vi "LoadFunction.vi"(8 "No Error":errorcluster, 10 "Name":string, 11 "Handle [SDL_SharedObject *]":i64 format="%.0x") -> (0 "Error Out":errorcluster, 3 "Function Pointer":i64 format="%.0x")   [LabVIEW 2024, in "SDL3.lvlib" / "LoadSO.lvlib"]
doc: "<B>Summary</B>\nLook up the address of the named function in a shared object.\n\n<B>Remarks</B>\nThis function pointer is no longer valid after calling <B>SDL_UnloadObject()</B>.\n\nThis function can only look up C function names. Other languages may have name mangling and intrinsic language support that varies from compiler to compiler.\n\nMake sure you declare your function pointers with the same calling convention as the actual library function. Your code will crash mysteriously if you do not do this.\n\nIf the requested function doesn't exist, NULL is returned."
uses:
  LoadSO/LoadSO.lvlib
  Error/Error.lvlib
  Lib/SDL3-32.dll
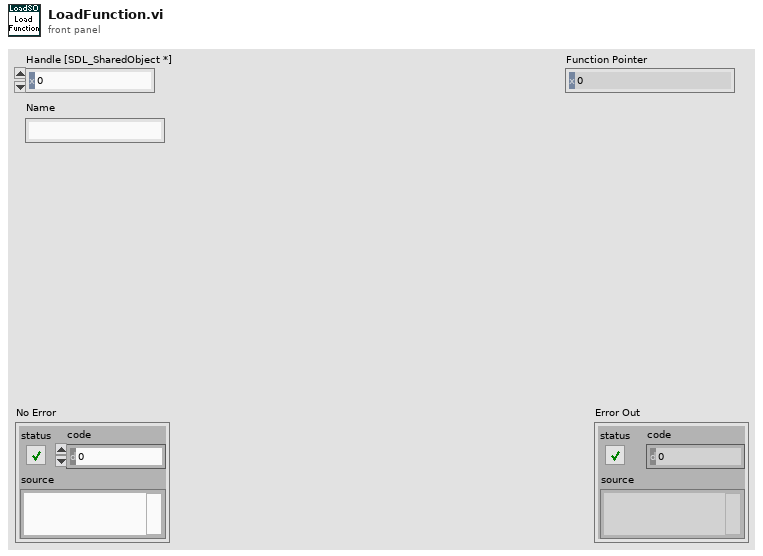
[diagram p1: front panel]
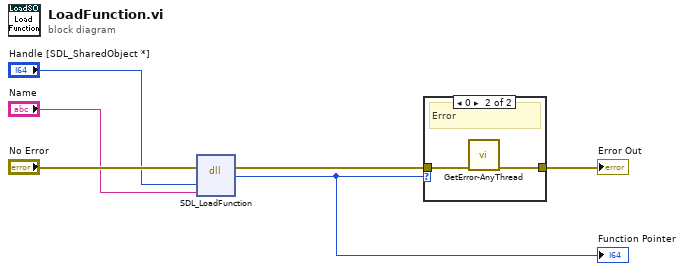
[diagram p0: block diagram]
diagram:
  n1 = dll-call lib="C:/Users/Thomas/Documents/Projects/LV-SDL3/Lib/SDL3-*.*" fn="SDL_LoadFunction"(error in="No Error", "handle"="Handle [SDL_SharedObject *]", "sofile"="Name") -> (error out=w4:errorcluster, "return type"=w1:i64)  [unwired: 4 in, 1 out]
  "Function Pointer" <- w1
  n2 = case shown="0" w1 {
    tunnel: w4 -> [w7 w9]
    tunnel: [w7 w8] -> w5
    frame Default {
      # "Ok"
    }
    frame 0 {
      # "Error"
      n3 = call "GetError-AnyThread.vi"("No Error"=w9) -> ("Error Out"=w8:errorcluster)  [unwired: 10 in]
    }
  }
  "Error Out" <- w5
